vi "NorStr2HexStr_Display.vi"(10 "Normal Display":string) -> (1 "Hex Display":string)   [LabVIEW 2017]
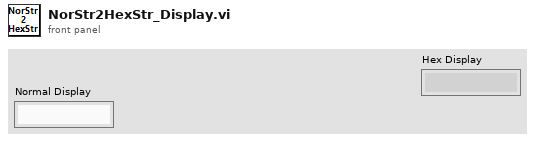
[diagram p1: front panel]
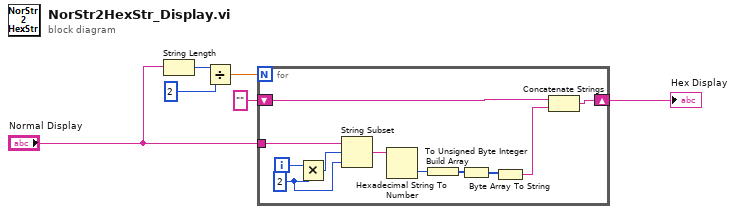
[diagram p0: block diagram]
diagram:
  n1 = String Length(string="Normal Display") -> (length=w6:i32)
  n2 = Divide(x=w6, y=2) -> (x/y=w4:dbl)
  n3 = for {
    N: w4 -> [_]
    shift-right: [w16] -> w1
    shift-left: "" -> [w17]
    tunnel: "Normal Display" -> [w15]
    i -> [w14]
    w7 = 2 ("y")
    n4 = Multiply(x=w14, y=w7) -> (x*y=w13:i32)
    n5 = String Subset(string=w15, offset (0)=w13, length (rest)=w7) -> (substring=w12:string)
    n6 = Hexadecimal String To Number(string=w12) -> (number=w11:u32)  [unwired: 2 in, 1 out]
    n7 = Build Array(w11) -> (w10:u32[])
    n8 = To Unsigned Byte Integer(number=w10) -> (unsigned 8bit integer=w9:u8[])
    n9 = Byte Array To String(unsigned byte array=w9) -> (string=w8:string)
    n10 = Concatenate Strings(w17, w8) -> (w16:string)
  }
  "Hex Display" <- w1
